vi "Read Data Server.vi"(8 "error in (no error)":errorcluster, 11 "veristand in":refnum<class "veristand-grpc.lvclass">) -> (0 "error out":errorcluster, 2 "veristand-grpc_server.lvlib:Data Server.lvclass":refnum<class "Data Server.lvclass">, 3 "veristand out":refnum<class "veristand-grpc.lvclass">)   [LabVIEW 2020, in "Veristandgrpc_server.lvlib" / "veristand-grpc.lvclass"]
uses:
  veristand-grpc.lvclass
  Data/Data Server.lvclass
  veristand-grpc.lvclass/veristand-grpc.ctl
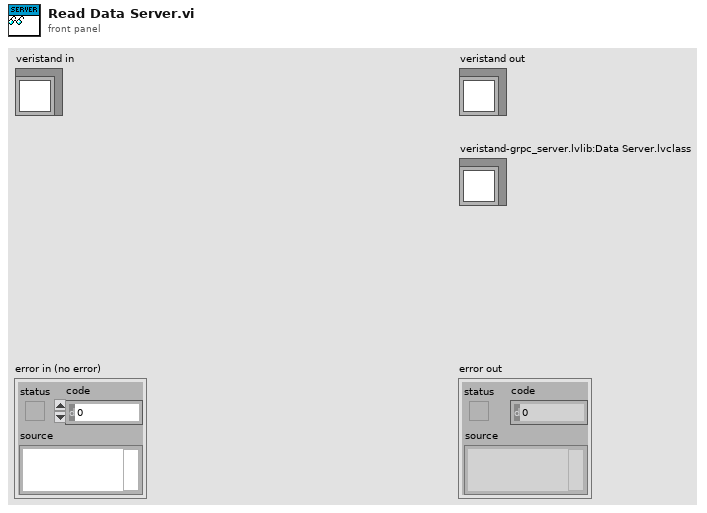
[diagram p1: front panel]
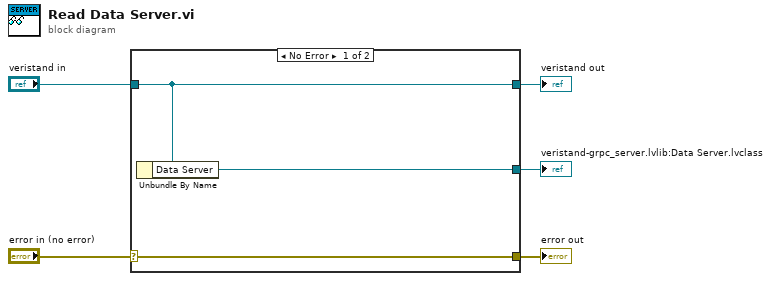
[diagram p0: block diagram]
diagram:
  n1 = case shown="No Error" "error in (no error)" {
    selector: "error in (no error)" -> [w8 w9]
    tunnel: [w8 w9] -> w4
    tunnel: [w7 w10] -> w2
    tunnel: "veristand in" -> [w7 w10]
    tunnel: [w6 _] -> w1
    frame No Error {
      n2 = Unbundle By Name(w7) -> ("Data Server"=w6:refnum<class "Data Server.lvclass">)
    }
    frame Error {
    }
  }
  "error out" <- w4
  "veristand out" <- w2
  "veristand-grpc_server.lvlib:Data Server.lvclass" <- w1
